vi "ReadFile.vi"(8 "error in (no error)":errorcluster, 11 "ReadOnly in":refnum<class "ReadOnly.lvclass">) -> (0 "error out":errorcluster, 2 "data":i32[](array[numeric]))   [LabVIEW 2021]
uses:
  Interfaces/ReadOnly/ReadOnly.lvclass
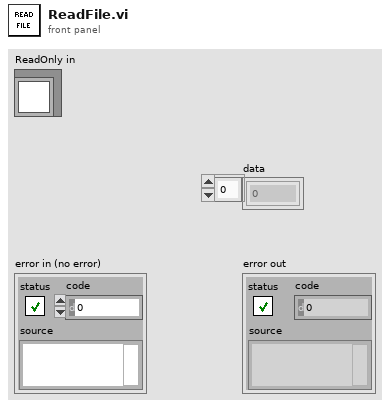
[diagram p1: front panel]
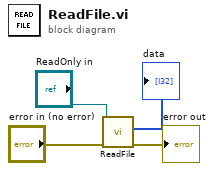
[diagram p0: block diagram]
diagram:
  n1 = call-dynamic "ReadFile.vi"("error in (no error)"="error in (no error)", "ReadOnly in"="ReadOnly in") -> ("error out"=→"error out":errorcluster, "data"=→"data":i32[])  [unwired: 8 in]
